vi "Create PrivateClass.vi"(5 "PrivateClass in":refnum<class "PrivateClass.lvclass">, 8 "error in (no error)":errorcluster, 11 "String":string) -> (0 "error out":errorcluster, 3 "PrivateClass":refnum<class "PrivateClass.lvclass">)   [LabVIEW 2017, in "TestLibrary.lvlib" / "PrivateClass.lvclass"]
uses:
  PrivateClass.lvclass
  PrivateClass.lvclass/PrivateClass.ctl
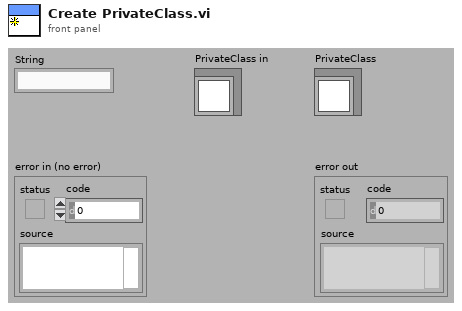
[diagram p1: front panel]
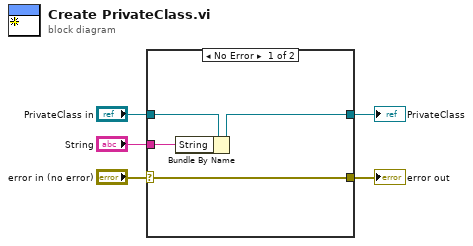
[diagram p0: block diagram]
diagram:
  n1 = case shown="No Error" "error in (no error)" {
    selector: "error in (no error)" -> [w9 w11]
    tunnel: [w9 w11] -> w4
    tunnel: [w7 w10] -> w2
    tunnel: "PrivateClass in" -> [w8 w10]
    tunnel: "String" -> [w6 _]
    frame No Error {
      n2 = Bundle By Name(cluster=w8, "String"=w6) -> (w7:refnum<class "PrivateClass.lvclass">)
    }
    frame Error {
    }
  }
  "error out" <- w4
  "PrivateClass" <- w2
